vi "GenerateDataSet.vi"(11 "Records":i32) -> (3 "DataGrid":string[][](array[string]))   [LabVIEW 2014, in "DataGrid.lvlib" / "DataGridView.lvclass"]
uses:
  DataGridView.lvclass
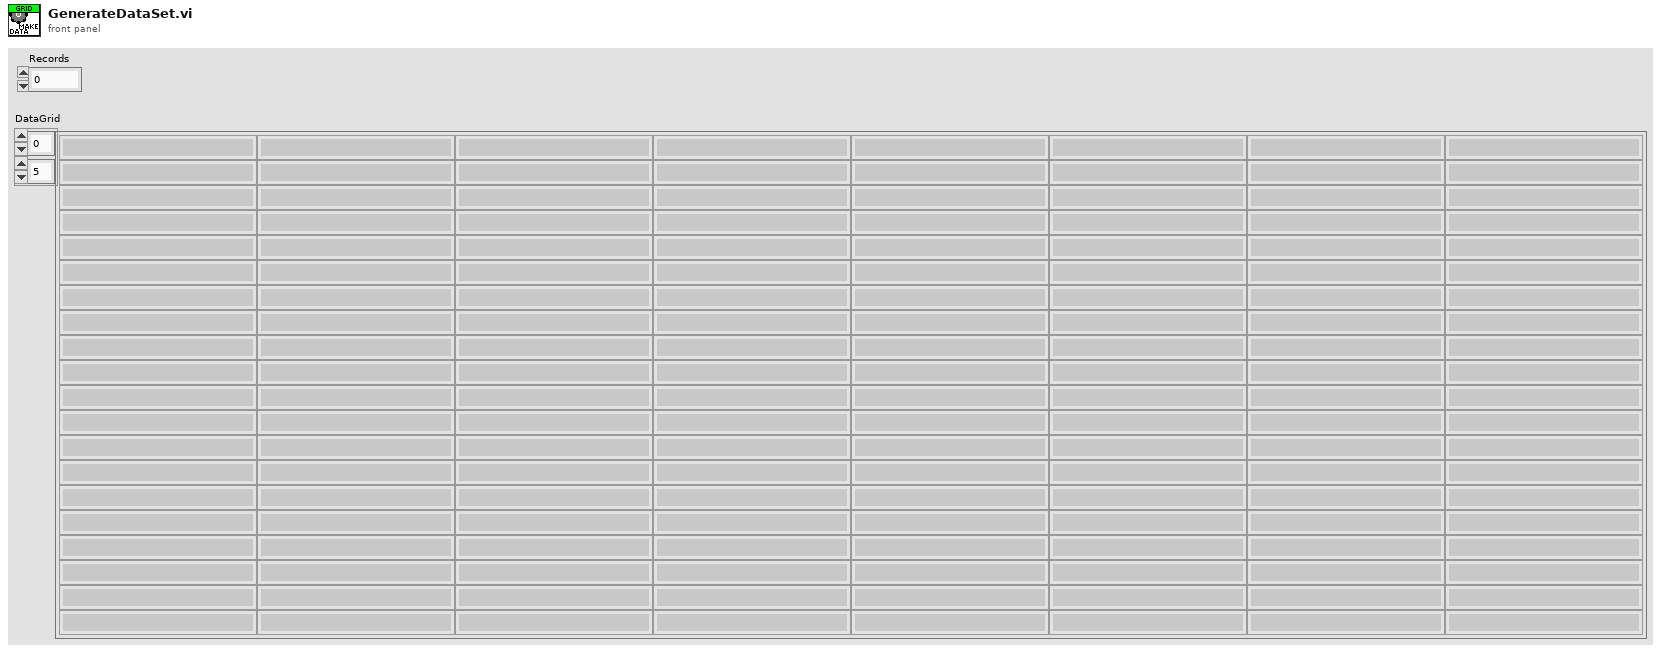
[diagram p1: front panel]
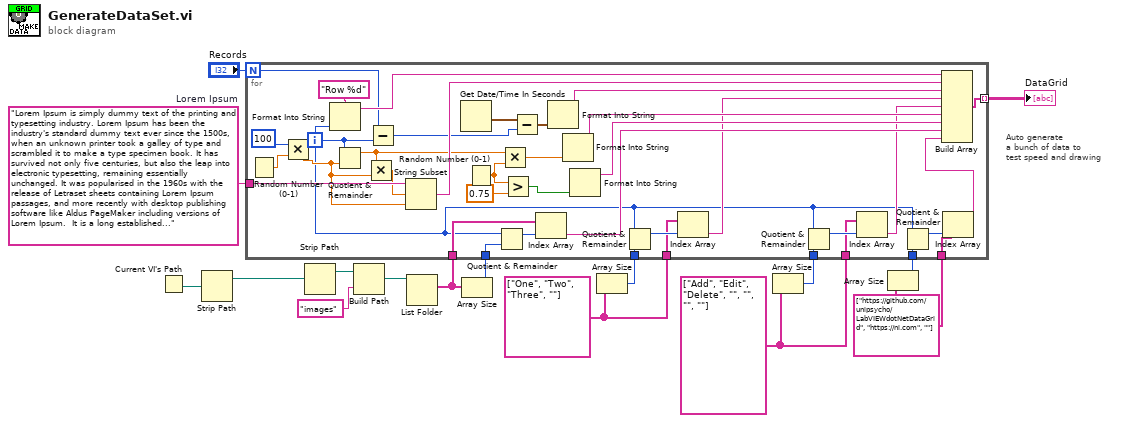
[diagram p0: block diagram]
diagram:
  w1 = string[] ["https://github.com/unipsycho/LabVIEWdotNetDataGrid", "https://ni.com", ""]
  w3 = string[] ["Add", "Edit", "Delete", "", "", "", ""]
  w5 = string[] ["One", "Two", "Three", ""]
  w10 = "Lorem Ipsum is simply dummy text of the printing and typesetting industry. Lorem Ipsum has been the industry's standard dummy text ever since the 1500s, when an unknown printer took a galley of type and scrambled it to make a type specimen book. It has survived not only five centuries, but also the leap into electronic typesetting, remaining essentially unchanged. It was popularised in the 1960s with the release of Letraset sheets containing Lorem Ipsum passages, and more recently with desktop publishing software like Aldus PageMaker including versions of Lorem Ipsum.  It is a long established fact that a reader will be distracted by the readable content of a page when looking at its layout. The point of using Lorem Ipsum is that it has a more-or-less normal distribution of letters, as opposed to using 'Content here, content here', making it look like readable English. Many desktop publishing packages and web page editors now use Lorem Ipsum as their default model text, and a search for 'lorem ipsum' will uncover many web sites still in their infancy. Various versions have evolved over the years, sometimes by accident, sometimes on purpose (injected humour and the like). Contrary to popular belief, Lorem Ipsum is not simply random text. It has roots in a piece of classical Latin literature from 45 BC, making it over 2000 years old. Richard McClintock, a Latin professor at Hampden-Sydney College in Virginia, looked up one of the more obscure Latin words, consectetur, from a Lorem Ipsum passage, and going through the cites of the word in classical literature, discovered the undoubtable source. Lorem Ipsum comes from sections 1.10.32 and 1.10.33 of \"de Finibus Bonorum et Malorum\" (The Extremes of Good and Evil) by Cicero, written in 45 BC. This book is a treatise on the theory of ethics, very popular during the Renaissance. The first line of Lorem Ipsum, \"Lorem ipsum dolor sit amet..\", comes from a line in section 1.10.32. The standard chunk of Lorem Ipsum used since the 1500s is reproduced below for those interested. Sections 1.10.32 and 1.10.33 from \"de Finibus Bonorum et Malorum\" by Cicero are also reproduced in their exact original form, accompanied by English versions from the 1914 translation by H. Rackham. There are many variations of passages of Lorem Ipsum available, but the majority have suffered alteration in some form, by injected humour, or randomised words which don't look even slightly believable. If you are going to use a passage of Lorem Ipsum, you need to be sure there isn't anything embarrassing hidden in the middle of text. All the Lorem Ipsum generators on the Internet tend to repeat predefined chunks as necessary, making this the first true generator on the Internet. It uses a dictionary of over 200 Latin words, combined with a handful of model sentence structures, to generate Lorem Ipsum which looks reasonable. The generated Lorem Ipsum is therefore always free from repetition, injected humour, or non-characteristic words etc."  # Lorem Ipsum
  # "Auto generate\na bunch of data to \ntest speed and drawing"
  n1 = Current VI's Path() -> (path=w8:path)
  n2 = Strip Path(path=w8) -> (stripped path=w7:path)  [unwired: 1 out]
  n3 = Strip Path(path=w7) -> (stripped path=w13:path)  [unwired: 1 out]
  n4 = Build Path(base path=w13, name or relative path="images") -> (appended path=w14:path)
  n5 = List Folder(path=w14) -> (filenames=w15:string[])  [unwired: 3 in, 3 out]
  n6 = Array Size(array=w15) -> (size(s)=w16:i32)
  n7 = Array Size(array=w5) -> (size(s)=w6:i32)
  n8 = Array Size(array=w3) -> (size(s)=w4:i32)
  n9 = Array Size(array=w1) -> (size(s)=w2:i32)
  n10 = for {
    N: "Records" -> [w47]
    tunnel: [w52] -> w9 mode=indexing
    tunnel: w10 -> [w51]
    tunnel: w15 -> [w35]
    tunnel: w16 -> [w36]
    tunnel: w5 -> [w31]
    tunnel: w6 -> [w30]
    tunnel: w4 -> [w27]
    tunnel: w3 -> [w26]
    tunnel: w2 -> [w21]
    tunnel: w1 -> [w20]
    i -> [w17]
    n11 = Random Number (0-1)() -> (number: 0 to 1=w24:dbl)
    n12 = Multiply(x=100 ("y"), y=w24) -> (x*y=w22:dbl)
    n13 = Format Into String(format string="Row %d", w17) -> (resulting string=w53:string)  [unwired: 2 in, 1 out]
    n14 = Quotient & Remainder(x=w17, y=w22) -> (x-y*floor(x/y)=w43:dbl)  [unwired: 1 out]
    n15 = Multiply(x=w43, y=w22) -> (x*y=w50:dbl)
    n16 = Subtract(x=w47, y=w17) -> (x-y=w46:i32)
    n17 = String Subset(string=w51, offset (0)=w50, length (rest)=w22) -> (substring=w49:string)
    n18 = Get Date/Time In Seconds() -> (seconds since 1Jan1904=w48:timestamp)
    n19 = Random Number (0-1)() -> (number: 0 to 1=w40:dbl)
    n20 = Quotient & Remainder(x=w17, y=w36) -> (x-y*floor(x/y)=w34:i32)  [unwired: 1 out]
    n21 = Multiply(x=w43, y=w40) -> (x*y=w42:dbl)
    n22 = Greater?(x=w40, y=0.75) -> (0:w38:bool)
    n23 = Subtract(x=w48, y=w46) -> (x-y=w45:timestamp)
    n24 = Index Array(array=w35, index=w34) -> (element=w33:string)
    n25 = Format Into String(w45) -> (resulting string=w44:string)  [unwired: 3 in, 1 out]
    n26 = Format Into String(w42) -> (resulting string=w41:string)  [unwired: 3 in, 1 out]
    n27 = Format Into String(w38) -> (resulting string=w37:string)  [unwired: 3 in, 1 out]
    n28 = Quotient & Remainder(x=w17, y=w30) -> (x-y*floor(x/y)=w32:i32)  [unwired: 1 out]
    n29 = Index Array(array=w31, index=w32) -> (element=w29:string)
    n30 = Quotient & Remainder(x=w17, y=w27) -> (x-y*floor(x/y)=w28:i32)  [unwired: 1 out]
    n31 = Index Array(array=w26, index=w28) -> (element=w25:string)
    n32 = Quotient & Remainder(x=w17, y=w21) -> (x-y*floor(x/y)=w19:i32)  [unwired: 1 out]
    n33 = Index Array(array=w20, index=w19) -> (element=w18:string)
    n34 = Build Array(w53, w49, w44, w29, w25, w41, w37, w33, w18) -> (w52:string[])
  }
  "DataGrid" <- w9
